vi "MPExxx_set_per.vi"(2 "error in (no error)":errorcluster, 3 "Set Period":dbl format="%.2f", 4 "VISA session":refnum<visa-resource-name>) -> (0 "error out":errorcluster, 1 "dup VISA session":refnum<visa-resource-name>)   [LabVIEW 2012]
doc: "This VI form sets the period of time that the power supply will remain in the state during auto sequence operation. The minimum unit for the period command is 10 msec. There are 3 reserved numbers associated with this command, namely: 0, 9998 and 9999. When a 0 is detected in auto sequence operation, the power supply will stop as if a stop command condition occurred. When a 9998 is detected, the following memory location will be zero. When 9999 is detected, the power supply will operate at that memory state indefinitely or until stop is commanded. The period's duration can be overridden by the using the start command to advance the memory to the next state or the stop command to stop the power supply."
uses:
  MPExxx Globals.gbl
panel:
  # "MAGNA-POWER"
  # "Electronics"
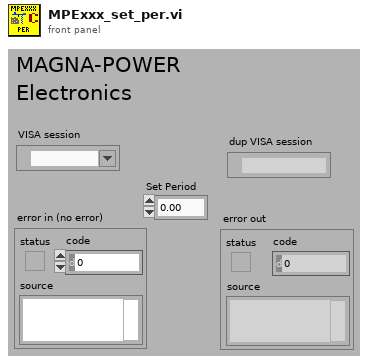
[diagram p1: front panel]
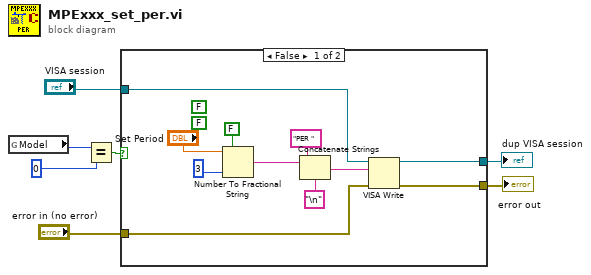
[diagram p0: block diagram]
diagram:
  n1 = global read "MPExxx Globals.gbl" "Model"() -> (w5:u8)
  n2 = Equal?(x=w5, y=0) -> (x = y?=w7:bool)
  n3 = case shown="False" w7 {
    tunnel: [w11 w20] -> w4
    tunnel: [w10 w19] -> w3
    tunnel: "VISA session" -> [w9 w20]
    tunnel: "error in (no error)" -> [w8 w19]
    frame False {
      (unwired) FALSE ("use system decimal point (T)")
      (unwired) FALSE ("use system decimal point (T)")
      n4 = Number To Fractional String(use system decimal point (T)=FALSE, number="Set Period", precision (6)=3) -> (F-format string=w17:string)  [unwired: 1 in]
      n5 = Concatenate Strings("PER ", w17, "\n") -> (w13:string)
      n6 = VISA Write(VISA resource name=w9, write buffer=w13, error in (no error)=w8) -> (VISA resource name out=w11:refnum<visa-resource-name>, error out=w10:errorcluster)  [unwired: 1 out]
    }
    frame True {
    }
  }
  "error out" <- w3
  "dup VISA session" <- w4
